vi "PacketExtract.vi"(2 "error in":errorcluster, 3 "Byte Array":u8[](array[numeric]), 4 "Input Message":T1={"Timestamp(4)"=0, "Sequence(4)"=0, "JY61ACC(2)"=[], "JY61GRY(3)"=[], "JY61AGL(3)"=[], "GY52ACC(2)"=[], "GY52GRY(3)"=[], "ADC1(3)"=[], "ADC2(3)"=[], "LFT/RAT"="DIR"}) -> (0 "error out":errorcluster, 1 "Output Message":T1={"Timestamp(4)"=0, "Sequence(4)"=0, "JY61ACC(2)"=[], "JY61GRY(3)"=[], "JY61AGL(3)"=[], "GY52ACC(2)"=[], "GY52GRY(3)"=[], "ADC1(3)"=[], "ADC2(3)"=[], "LFT/RAT"="DIR"})   [LabVIEW 2014]
panel:
  out "Verified":bool=TRUE
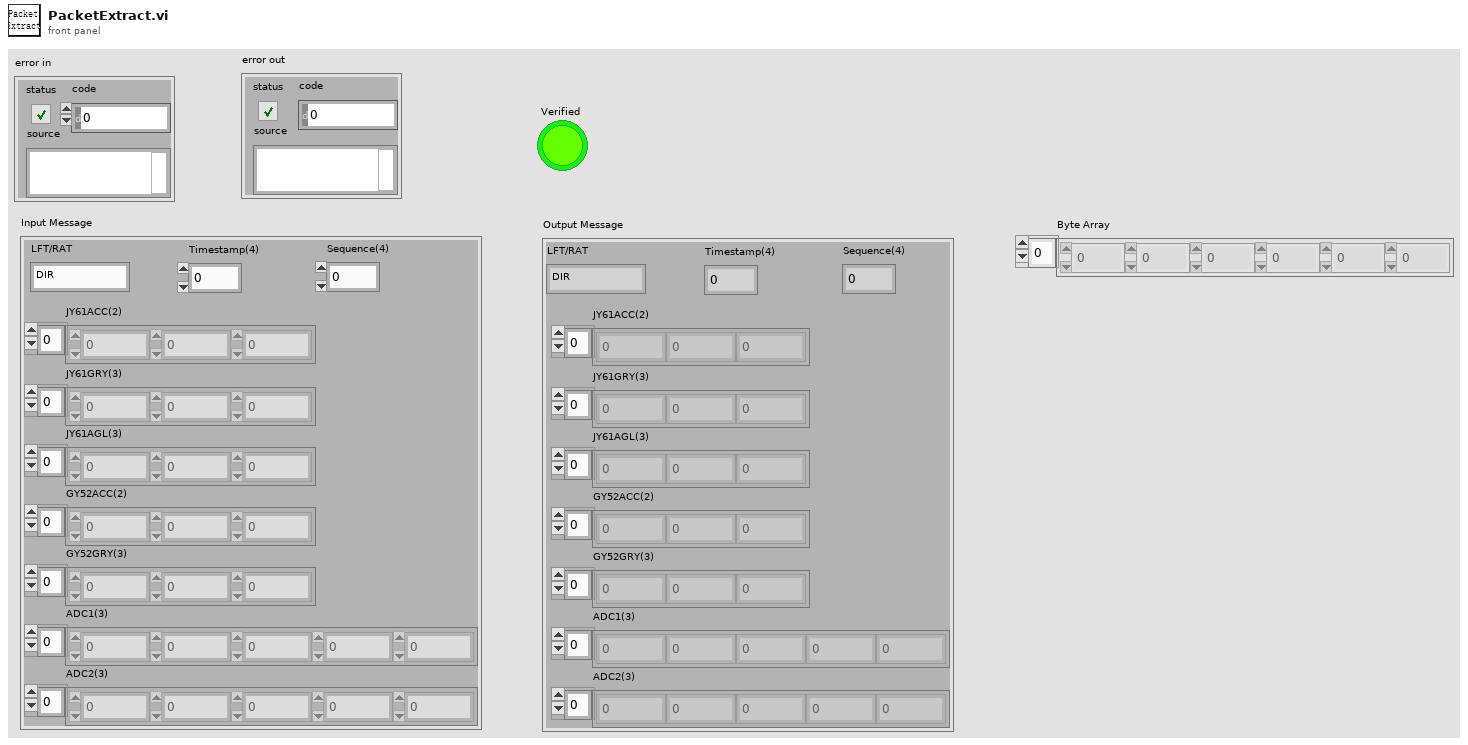
[diagram p1: front panel]
types:
  T1 = cluster{"Timestamp(4)":u32, "Sequence(4)":u32, "JY61ACC(2)":dbl[], "JY61GRY(3)":dbl[], "JY61AGL(3)":dbl[], "GY52ACC(2)":dbl[], "GY52GRY(3)":dbl[], "ADC1(3)":dbl[], "ADC2(3)":dbl[], "LFT/RAT":string}
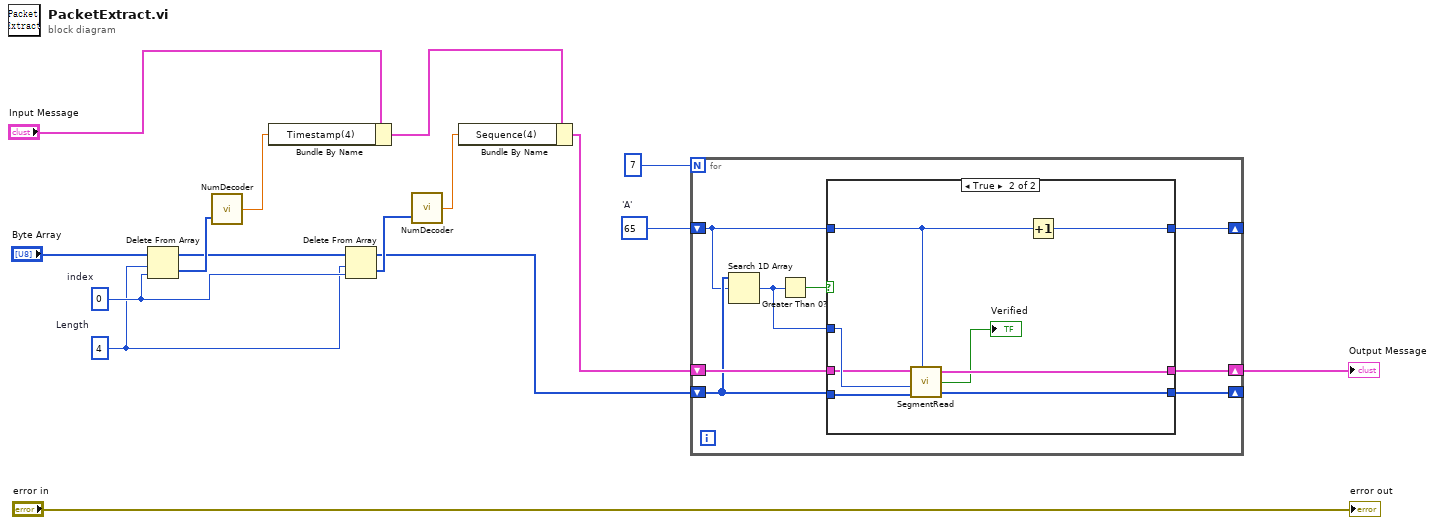
[diagram p0: block diagram]
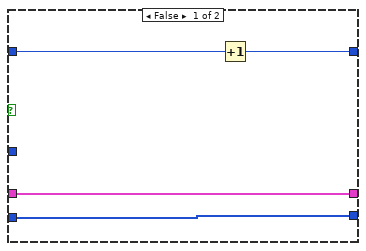
[diagram p2: hidden frame]
diagram:
  w10 = u8 65  # 'A'
  w4 = 0  # index
  w3 = 4  # Length
  n1 = Delete From Array(array="Byte Array", length=w3, index=w4) -> (deleted portion=w6:u8[], array with subset deleted=w5:u8[])
  n2 = call "NumDecoder.vi"("Byte Array"=w6) -> ("Number"=w14:dbl)  [unwired: 1 in]
  n3 = Bundle By Name(cluster="Input Message", "Timestamp(4)"=w14) -> (w16:T1)
  n4 = Delete From Array(array=w5, length=w3, index=w4) -> (deleted portion=w2:u8[], array with subset deleted=w1:u8[])
  n5 = call "NumDecoder.vi"("Byte Array"=w2) -> ("Number"=w12:dbl)  [unwired: 1 in]
  n6 = Bundle By Name(cluster=w16, "Sequence(4)"=w12) -> (w9:T1)
  n7 = for {
    N: 7 -> [_]
    shift-right: [w24] -> _
    shift-left: w1 -> [w21]
    shift-right: [w18] -> _
    shift-left: w10 -> [w20]
    shift-right: [w23] -> w8
    shift-left: w9 -> [w22]
    n8 = Search 1D Array(1D array=w21, element=w20) -> (index of element=w17:i32)  [unwired: 1 in]
    n9 = Greater Than 0?(x=w17) -> (x > 0?=w19:bool)
    n10 = case shown="True" w19 {
      tunnel: [w28 w35] -> w24
      tunnel: w21 -> [w28 w36]
      tunnel: [w27 w32] -> w23
      tunnel: w22 -> [w27 w33]
      tunnel: [w25 w30] -> w18
      tunnel: w20 -> [w26 w31]
      tunnel: w17 -> [_ w34]
      frame False {
        n11 = Increment(x=w26) -> (x+1=w25:u8)
      }
      frame True {
        n12 = call "SegmentRead.vi"("Input Message"=w33, "index"=w34, "Input Byte Array"=w36, "Char"=w31) -> ("Output Message"=w32:T1, "Verified"=→"Verified":bool, "Output Byte Array"=w35:u8[])  [unwired: 1 in]
        n13 = Increment(x=w31) -> (x+1=w30:u8)
      }
    }
  }
  "Output Message" <- w8
  "error out" <- "error in"
